vi "Sensor_Reads.vi"() -> ()   [LabVIEW 2019]
uses:
  M14 Hardware/Flywheel/M14_Flywheel_Hardware_Globals.vi
  M14 Hardware/Drive/M14_Drive_Hardware_Globals.vi
  M14 Hardware/Spindexer/M14_Hardware_Spindexer_Globals.vi
  M14 Hardware/New Magazine/New_Magazine_Hardware_Globals.vi
  M14 Hardware/Turret/M14 Turret_Hardware_Globals.vi
  M14 Hardware/Control Panel/M14_Control_Panel_Globals.vi
  Subsystems/Sensing/Sensor_Values.vi
  <vilib>/Rock Robotics/WPI/ThirdParty/Phoenix-LabVIEW/Motor Controller/Get/CTRE_Phoenix_MotorController_GetSelectedSensorData.vi
  M14 Hardware/Sensors/IMU/M14_IMU_Hardware_Globals.vi
  M14 Hardware/Sensors/IRs & Limits/M14_IR&Limits_Hardware_Globals.vi
  <vilib>/Rock Robotics/WPI/ThirdParty/Phoenix-LabVIEW/Pigeon IMU/CTRE_PigeonIMU_GetYPR.vi
panel:
  out "Right_Drive_Position(feet)":dbl
  out "Left_Drive_Position(feet)":dbl
  in  "F":dbl=0.365
  in  "D":dbl
  in  "I":dbl
  in  "P":dbl
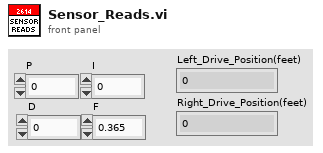
[diagram p1: front panel]
types:
  T1 = typedef "WPI_MotorControlDeviceRef.ctl" = cluster{"DeviceStatus":errorcluster, "Type":T2, "PWM":cluster{"PWM Channel":T3, "DeadBand":T4}, "CAN":cluster{"Device Number":u8, "SetOutput VI Ref":variant, "GetOutput VI Ref":variant, "Enable VI Ref":variant, "Disable VI Ref":variant, "Data":variant}, "Invert":bool, "DIO PWM":cluster{"PWM \"Enable\" Channel":T3, "DIOChannel":T5, "PWM Rate":dbl}}
  T2 = typedef "WPI_MotorControlType.ctl" = enum16{"PWM", "CAN", "DIO PWM"}
  T3 = typedef "FPGA_DIOPWMChannel.ctl" = enum8{"PWM 0", "PWM 1", "PWM 2", "PWM 3", "PWM 4", "PWM 5", "PWM 6", "PWM 7", "PWM 8", "PWM 9", "PWM MXP 0", "PWM MXP 1", "PWM MXP 2", "PWM MXP 3", "PWM MXP 4", "PWM MXP 5", "PWM MXP 6", "PWM MXP 7", "PWM MXP 8", "PWM MXP 9", "Invalid"}
  T4 = typedef "WPI_PWMDeadband.ctl" = cluster{"Name":string, "maxPositivePwm":i32, "minPositivePwm":i32, "centerPwm":i32, "maxNegativePwm":i32, "minNegativePwm":i32, "angularRange":u16}
  T5 = typedef "FPGA_DIOChannel.ctl" = enum8{"DIO 0", "DIO 1", "DIO 2", "DIO 3", "DIO 4", "DIO 5", "DIO 6", "DIO 7", "DIO 8", "DIO 9", "DIO MXP 0", "DIO MXP 1", "DIO MXP 2", "DIO MXP 3", "DIO MXP 4", "DIO MXP 5", "DIO MXP 6", "DIO MXP 7", "DIO MXP 8", "DIO MXP 9", "DIO MXP 10", "DIO MXP 11", "DIO MXP 12", "DIO MXP 13", "DIO MXP 14", "DIO MXP 15", "SPI Port CS1", "SPI Port CS2", "SPI Port CS3", "SPI Port MISO", "SPI Port MOSI", "Invalid"}
  T6 = typedef "CTRE_PigeonIMU_DeviceRef.ctl" = cluster{"DeviceStatus":errorcluster, "Device Number":u8, "Type":T7, "Device ID":u32, "Handle":u64, "UsageFrame":u32, "Library Path":path}
  T7 = typedef "CTRE_PigeonIMU_ConnectionType.ctl" = u32
  T8 = typedef "WPI_DigitalInputDevRef.ctl" = cluster{"DevStatus":errorcluster, "DIO Channel":T5}
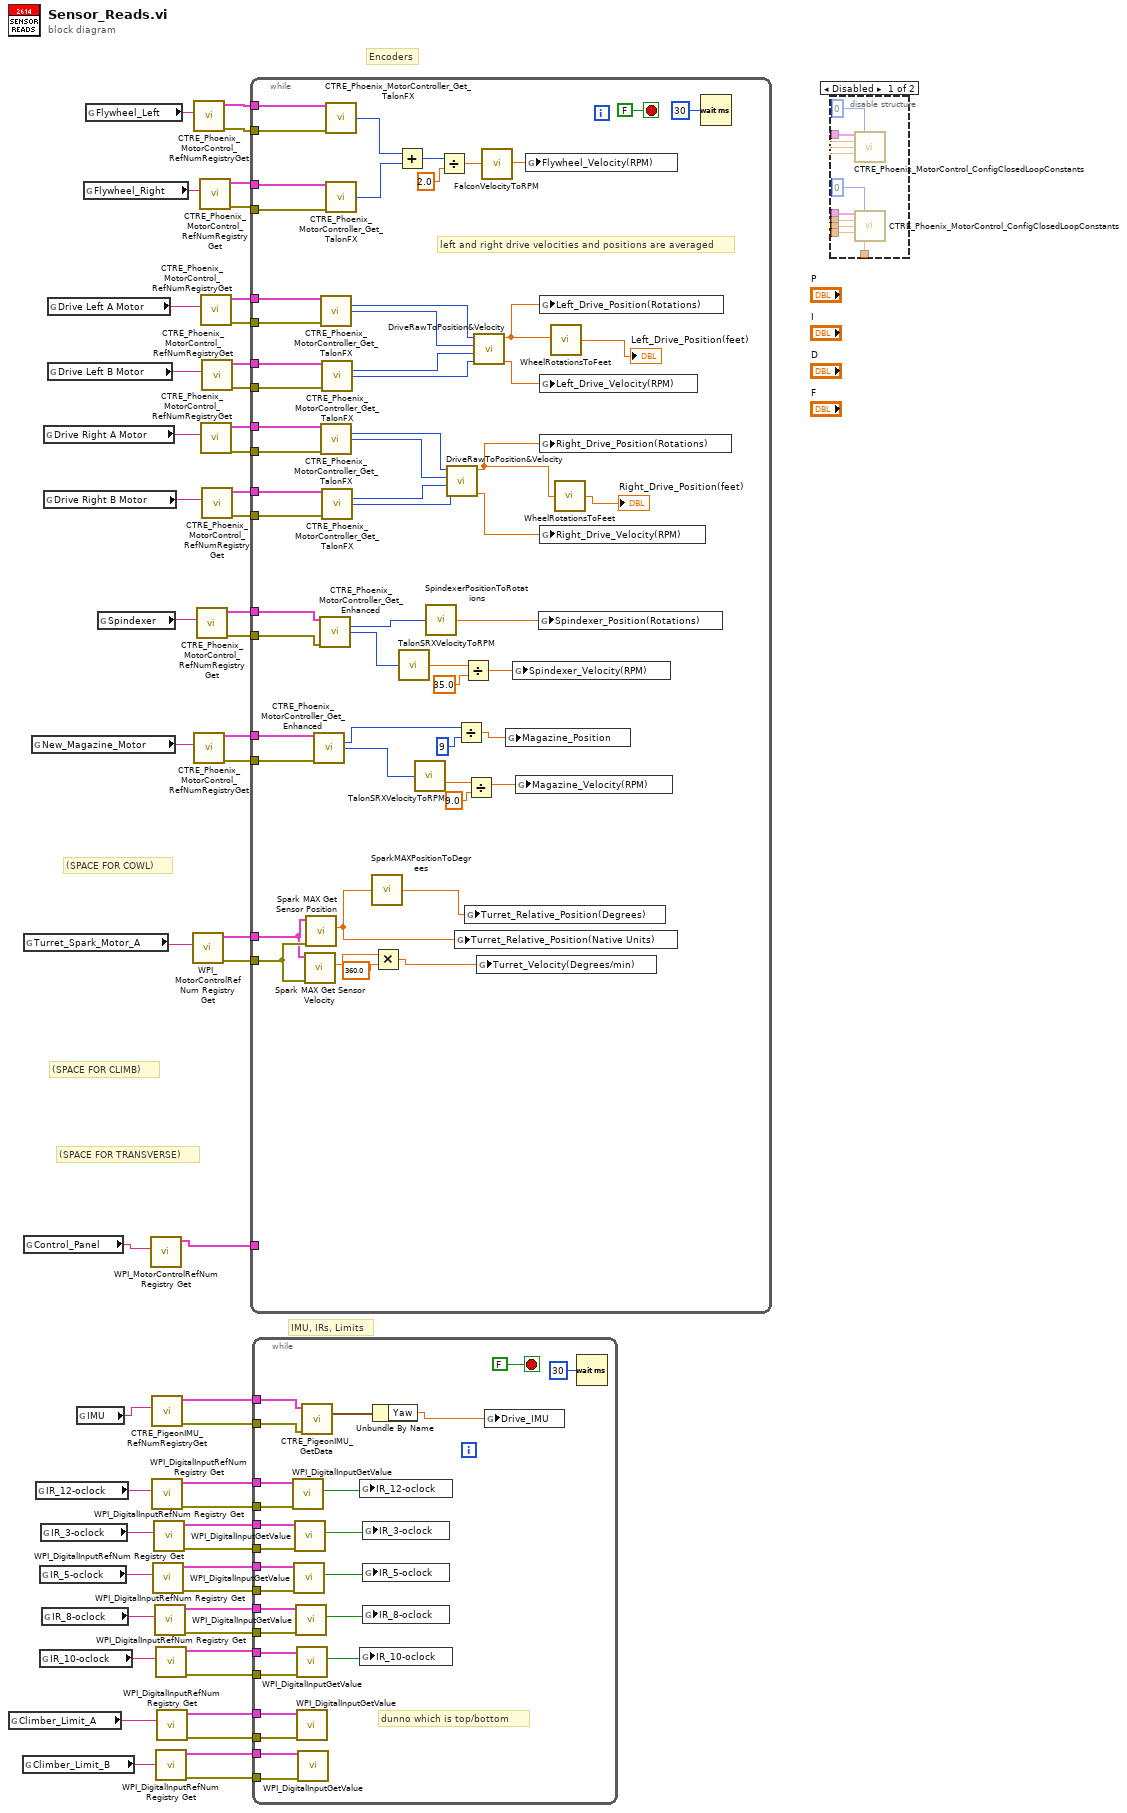
[diagram p0: block diagram]
diagram:
  # "IMU, IRs, Limits"
  # "(SPACE FOR TRANSVERSE)"
  # "(SPACE FOR CLIMB)"
  # "(SPACE FOR COWL)"
  # "Encoders"
  n1 = global read "M14_IR&Limits_Hardware_Globals.vi" "Climber_Limit_A"() -> (w6:string)
  n2 = global read "M14_IR&Limits_Hardware_Globals.vi" "Climber_Limit_B"() -> (w5:string)
  n3 = global read "M14 Turret_Hardware_Globals.vi" "Turret_Spark_Motor_A"() -> (w35:string)
  n4 = global read "M14_Control_Panel_Globals.vi" "Control_Panel"() -> (w33:string)
  n5 = global read "New_Magazine_Hardware_Globals.vi" "New_Magazine_Motor"() -> (w37:string)
  n6 = global read "M14_IR&Limits_Hardware_Globals.vi" "IR_12-oclock"() -> (w19:string)
  n7 = global read "M14_IR&Limits_Hardware_Globals.vi" "IR_5-oclock"() -> (w13:string)
  n8 = global read "M14_IR&Limits_Hardware_Globals.vi" "IR_10-oclock"() -> (w7:string)
  n9 = global read "M14_IR&Limits_Hardware_Globals.vi" "IR_3-oclock"() -> (w18:string)
  n10 = global read "M14_IR&Limits_Hardware_Globals.vi" "IR_8-oclock"() -> (w12:string)
  n11 = global read "M14_Drive_Hardware_Globals.vi" "Drive Right A Motor"() -> (w40:string)
  n12 = global read "M14_Drive_Hardware_Globals.vi" "Drive Right B Motor"() -> (w43:string)
  n13 = global read "M14_Drive_Hardware_Globals.vi" "Drive Left A Motor"() -> (w47:string)
  n14 = global read "M14_Drive_Hardware_Globals.vi" "Drive Left B Motor"() -> (w44:string)
  n15 = global read "M14_IMU_Hardware_Globals.vi" "IMU"() -> (w31:string)
  n16 = global read "M14_Flywheel_Hardware_Globals.vi" "Flywheel_Right"() -> (w52:string)
  n17 = global read "M14_Flywheel_Hardware_Globals.vi" "Flywheel_Left"() -> (w53:string)
  n18 = global read "M14_Hardware_Spindexer_Globals.vi" "Spindexer"() -> (w39:string)
  n19 = call <vilib>:"WPI_MotorControlRefNum Registry Get.vi"("refnum name"=w33) -> ("MotorControlDevRef"=w32:T1)  [unwired: 9 in, 1 out]
  n20 = call <vilib>:"CTRE_PigeonIMU_RefNumRegistryGet.vi"("refnum name"=w31) -> ("error out"=w22:errorcluster, "PigeonIMUDevRef"=w30:T6)  [unwired: 9 in]
  n21 = call <vilib>:"WPI_DigitalInputRefNum Registry Get.vi"("refnum name"=w19) -> ("error out"=w20:errorcluster, "DigitalInputDevRef"=w21:T8)  [unwired: 9 in]
  n22 = call <vilib>:"WPI_DigitalInputRefNum Registry Get.vi"("refnum name"=w13) -> ("error out"=w14:errorcluster, "DigitalInputDevRef"=w15:T8)  [unwired: 9 in]
  n23 = call <vilib>:"WPI_DigitalInputRefNum Registry Get.vi"("refnum name"=w18) -> ("error out"=w17:errorcluster, "DigitalInputDevRef"=w16:T8)  [unwired: 9 in]
  n24 = call <vilib>:"WPI_DigitalInputRefNum Registry Get.vi"("refnum name"=w12) -> ("error out"=w11:errorcluster, "DigitalInputDevRef"=w10:T8)  [unwired: 9 in]
  n25 = call <vilib>:"WPI_DigitalInputRefNum Registry Get.vi"("refnum name"=w7) -> ("error out"=w8:errorcluster, "DigitalInputDevRef"=w9:T8)  [unwired: 9 in]
  n26 = call <vilib>:"WPI_DigitalInputRefNum Registry Get.vi"("refnum name"=w5) -> ("error out"=w1:errorcluster, "DigitalInputDevRef"=w2:T8)  [unwired: 9 in]
  n27 = call <vilib>:"WPI_DigitalInputRefNum Registry Get.vi"("refnum name"=w6) -> ("error out"=w3:errorcluster, "DigitalInputDevRef"=w4:T8)  [unwired: 9 in]
  n28 = call <vilib>:"WPI_MotorControlRefNum Registry Get.vi"("refnum name"=w35) -> ("error out"=w23:errorcluster, "MotorControlDevRef"=w34:T1)  [unwired: 9 in]
  n29 = call <vilib>:"CTRE_Phoenix_MotorControl_RefNumRegistryGet.vi"("refnum name"=w53) -> ("error out"=w50:errorcluster, "PhoenixMotorControlDevRef"=w51:T1)  [unwired: 9 in]
  n30 = call <vilib>:"CTRE_Phoenix_MotorControl_RefNumRegistryGet.vi"("refnum name"=w37) -> ("error out"=w24:errorcluster, "PhoenixMotorControlDevRef"=w36:T1)  [unwired: 9 in]
  n31 = call <vilib>:"CTRE_Phoenix_MotorControl_RefNumRegistryGet.vi"("refnum name"=w39) -> ("error out"=w25:errorcluster, "PhoenixMotorControlDevRef"=w38:T1)  [unwired: 9 in]
  n32 = call <vilib>:"CTRE_Phoenix_MotorControl_RefNumRegistryGet.vi"("refnum name"=w52) -> ("error out"=w48:errorcluster, "PhoenixMotorControlDevRef"=w49:T1)  [unwired: 9 in]
  n33 = call <vilib>:"CTRE_Phoenix_MotorControl_RefNumRegistryGet.vi"("refnum name"=w47) -> ("error out"=w29:errorcluster, "PhoenixMotorControlDevRef"=w46:T1)  [unwired: 9 in]
  n34 = call <vilib>:"CTRE_Phoenix_MotorControl_RefNumRegistryGet.vi"("refnum name"=w40) -> ("error out"=w27:errorcluster, "PhoenixMotorControlDevRef"=w41:T1)  [unwired: 9 in]
  n35 = call <vilib>:"CTRE_Phoenix_MotorControl_RefNumRegistryGet.vi"("refnum name"=w44) -> ("error out"=w28:errorcluster, "PhoenixMotorControlDevRef"=w45:T1)  [unwired: 9 in]
  n36 = call <vilib>:"CTRE_Phoenix_MotorControl_RefNumRegistryGet.vi"("refnum name"=w43) -> ("error out"=w26:errorcluster, "PhoenixMotorControlDevRef"=w42:T1)  [unwired: 9 in]
  n37 = while {
    tunnel: w51 -> [w109]
    tunnel: w50 -> [w108]
    tunnel: w49 -> [w107]
    tunnel: w48 -> [w106]
    tunnel: w46 -> [w105]
    tunnel: w45 -> [w104]
    tunnel: w41 -> [w102]
    tunnel: w42 -> [w103]
    tunnel: w38 -> [w92]
    tunnel: w36 -> [w89]
    tunnel: w34 -> [w70]
    tunnel: w32 -> [_]
    tunnel: w29 -> [w77]
    tunnel: w28 -> [w76]
    tunnel: w27 -> [w75]
    tunnel: w26 -> [w74]
    tunnel: w25 -> [w73]
    tunnel: w24 -> [w72]
    tunnel: w23 -> [w71]
    stop <- FALSE stop-if-true
    # "left and right drive velocities and positions are averaged"
    n38 = call <vilib>:"Spark MAX Get Sensor Velocity.vi"("error in (no error)"=w71, "MotorControlDevRef in"=w70) -> ("Sensor Velocity"=w61:dbl)  [unwired: 6 in, 3 out]
    n39 = call <vilib>:"Spark MAX Get Sensor Position.vi"("error in (no error)"=w71, "MotorControlDevRef in"=w70) -> ("Sensor Position"=w58:dbl)  [unwired: 6 in, 3 out]
    n40 = call-poly <vilib>:"CTRE_Phoenix_MotorController_Get_Enhanced.vi"("PhoenixMotorControlDevRef"=w89, "error in"=w72) -> ("Position (Raw Sensor Units)"=w85:i32, "Velocity (Raw Sensor Units per 100 ms)"=w88:i32)  [unwired: 10 in, 2 out]
    n41 = call-poly <vilib>:"CTRE_Phoenix_MotorController_Get_Enhanced.vi"("PhoenixMotorControlDevRef"=w92, "error in"=w73) -> ("Position (Raw Sensor Units)"=w90:i32, "Velocity (Raw Sensor Units per 100 ms)"=w91:i32)  [unwired: 10 in, 2 out]
    n42 = call-poly <vilib>:"CTRE_Phoenix_MotorController_Get_TalonFX.vi"("PhoenixMotorControlDevRef"=w105, "error in"=w77) -> ("Position (Raw Sensor Units)"=w94:i32, "Velocity (Raw Sensor Units per 100 ms)"=w101:i32)  [unwired: 10 in, 2 out]
    n43 = call-poly <vilib>:"CTRE_Phoenix_MotorController_Get_TalonFX.vi"("PhoenixMotorControlDevRef"=w102, "error in"=w75) -> ("Position (Raw Sensor Units)"=w67:i32, "Velocity (Raw Sensor Units per 100 ms)"=w66:i32)  [unwired: 10 in, 2 out]
    n44 = call-poly <vilib>:"CTRE_Phoenix_MotorController_Get_TalonFX.vi"("PhoenixMotorControlDevRef"=w104, "error in"=w76) -> ("Position (Raw Sensor Units)"=w93:i32, "Velocity (Raw Sensor Units per 100 ms)"=w69:i32)  [unwired: 10 in, 2 out]
    n45 = call-poly <vilib>:"CTRE_Phoenix_MotorController_Get_TalonFX.vi"("PhoenixMotorControlDevRef"=w103, "error in"=w74) -> ("Position (Raw Sensor Units)"=w65:i32, "Velocity (Raw Sensor Units per 100 ms)"=w64:i32)  [unwired: 10 in, 2 out]
    n46 = call-poly <vilib>:"CTRE_Phoenix_MotorController_Get_TalonFX.vi"("PhoenixMotorControlDevRef"=w109, "error in"=w108) -> ("Velocity (Raw Sensor Units per 100 ms)"=w97:i32)  [unwired: 10 in, 3 out]
    n47 = call-poly <vilib>:"CTRE_Phoenix_MotorController_Get_TalonFX.vi"("PhoenixMotorControlDevRef"=w107, "error in"=w106) -> ("Velocity (Raw Sensor Units per 100 ms)"=w96:i32)  [unwired: 10 in, 3 out]
    n48 = call "SparkMAXPositionToDegrees.vi"("Sensor Position"=w58) -> ("degrees"=w59:dbl)  [unwired: 4 in]
    n49 = Multiply(x=w61, y=360.0) -> (x*y=w62:dbl)
    n50 = Add(x=w97, y=w96) -> (x+y=w98:i32)
    n51 = call "TalonSRXVelocityToRPM.vi"("Velocity (Raw Sensor Units per 100 ms)"=w91) -> ("RPM"=w81:dbl)  [unwired: 4 in]
    n52 = call "TalonSRXVelocityToRPM.vi"("Velocity (Raw Sensor Units per 100 ms)"=w88) -> ("RPM"=w87:dbl)  [unwired: 4 in]
    n53 = call "SpindexerPositionToRotations.vi"("Position (Raw Sensor Units)"=w90) -> ("Numeric"=w78:dbl)  [unwired: 4 in]
    n54 = Divide(x=w98, y=2.0) -> (x/y=w95:dbl)
    n55 = call "DriveRawToPosition&Velocity.vi"("Velocity (Raw Sensor Units per 100 ms) B"=w64, "Position (Raw Sensor Units) B"=w65, "Velocity (Raw Sensor Units per 100 ms) A"=w66, "Position (Raw Sensor Units) A"=w67) -> ("Velocity"=w63:dbl, "Position"=w55:dbl)  [unwired: 6 in]
    n56 = global write "Sensor_Values.vi" "Turret_Relative_Position(Native Units)"(w58) -> ()
    n57 = Divide(x=w85, y=9) -> (x/y=w86:dbl)
    n58 = Divide(x=w81, y=35.0) -> (x/y=w79:dbl)
    n59 = global write "Sensor_Values.vi" "Turret_Relative_Position(Degrees)"(w59) -> ()
    n60 = Divide(x=w87, y=9.0) -> (x/y=w83:dbl)
    n61 = call "DriveRawToPosition&Velocity.vi"("Velocity (Raw Sensor Units per 100 ms) B"=w69, "Position (Raw Sensor Units) B"=w93, "Velocity (Raw Sensor Units per 100 ms) A"=w101, "Position (Raw Sensor Units) A"=w94) -> ("Velocity"=w68:dbl, "Position"=w57:dbl)  [unwired: 6 in]
    n62 = global write "Sensor_Values.vi" "Turret_Velocity(Degrees/min)"(w62) -> ()
    n63 = call "FalconVelocityToRPM.vi"("raw sensor units / 100 ms"=w95) -> ("RPM"=w100:dbl)  [unwired: 4 in]
    n64 = global write "Sensor_Values.vi" "Magazine_Position"(w86) -> ()
    n65 = global write "Sensor_Values.vi" "Spindexer_Velocity(RPM)"(w79) -> ()
    n66 = global write "Sensor_Values.vi" "Magazine_Velocity(RPM)"(w83) -> ()
    n67 = global write "Sensor_Values.vi" "Flywheel_Velocity(RPM)"(w100) -> ()
    n68 = global write "Sensor_Values.vi" "Spindexer_Position(Rotations)"(w78) -> ()
    n69 = global write "Sensor_Values.vi" "Left_Drive_Position(Rotations)"(w57) -> ()
    n70 = global write "Sensor_Values.vi" "Left_Drive_Velocity(RPM)"(w68) -> ()
    n71 = global write "Sensor_Values.vi" "Right_Drive_Position(Rotations)"(w55) -> ()
    n72 = global write "Sensor_Values.vi" "Right_Drive_Velocity(RPM)"(w63) -> ()
    n73 = call "WheelRotationsToFeet.vi"("rotations"=w57) -> ("feet"=→"Left_Drive_Position(feet)":dbl)  [unwired: 4 in]
    n74 = call "WheelRotationsToFeet.vi"("rotations"=w55) -> ("feet"=→"Right_Drive_Position(feet)":dbl)  [unwired: 4 in]
    n75 = Wait (ms)(milliseconds to wait=u32 30) -> ()  [unwired: 1 out]
  }
  n76 = while {
    tunnel: w30 -> [w135]
    tunnel: w22 -> [w134]
    tunnel: w21 -> [w130]
    tunnel: w20 -> [w129]
    tunnel: w16 -> [w127]
    tunnel: w17 -> [w128]
    tunnel: w15 -> [w126]
    tunnel: w14 -> [w125]
    tunnel: w10 -> [w123]
    tunnel: w11 -> [w124]
    tunnel: w9 -> [w122]
    tunnel: w8 -> [w121]
    tunnel: w4 -> [w115]
    tunnel: w3 -> [w114]
    tunnel: w2 -> [w113]
    tunnel: w1 -> [w112]
    stop <- FALSE stop-if-true
    # "dunno which is top/bottom"
    n77 = call <vilib>:"WPI_DigitalInputGetValue.vi"("error in (no error)"=w129, "DigitalInputDevRef"=w130) -> ("Value"=w120:bool)  [unwired: 7 in, 2 out]
    n78 = call <vilib>:"WPI_DigitalInputGetValue.vi"("error in (no error)"=w125, "DigitalInputDevRef"=w126) -> ("Value"=w118:bool)  [unwired: 7 in, 2 out]
    n79 = call <vilib>:"WPI_DigitalInputGetValue.vi"("error in (no error)"=w128, "DigitalInputDevRef"=w127) -> ("Value"=w119:bool)  [unwired: 7 in, 2 out]
    n80 = call <vilib>:"WPI_DigitalInputGetValue.vi"("error in (no error)"=w124, "DigitalInputDevRef"=w123) -> ("Value"=w117:bool)  [unwired: 7 in, 2 out]
    n81 = call <vilib>:"WPI_DigitalInputGetValue.vi"("error in (no error)"=w121, "DigitalInputDevRef"=w122) -> ("Value"=w116:bool)  [unwired: 7 in, 2 out]
    n82 = call <vilib>:"WPI_DigitalInputGetValue.vi"("error in (no error)"=w114, "DigitalInputDevRef"=w115) -> ()  [unwired: 7 in, 3 out]
    n83 = call <vilib>:"WPI_DigitalInputGetValue.vi"("error in (no error)"=w112, "DigitalInputDevRef"=w113) -> ()  [unwired: 7 in, 3 out]
    n84 = call-poly <vilib>:"CTRE_PigeonIMU_GetData.vi"("error in (no error)"=w134, "PigeonIMUDevRef"=w135) -> ("Yaw Pitch Roll"=w133:cluster{"Yaw":dbl, "Pitch":dbl, "Roll":dbl})  [unwired: 7 in, 2 out]
    n85 = global write "Sensor_Values.vi" "IR_12-oclock"(w120) -> ()
    n86 = global write "Sensor_Values.vi" "IR_10-oclock"(w116) -> ()
    n87 = global write "Sensor_Values.vi" "IR_3-oclock"(w119) -> ()
    n88 = global write "Sensor_Values.vi" "IR_5-oclock"(w118) -> ()
    n89 = global write "Sensor_Values.vi" "IR_8-oclock"(w117) -> ()
    n90 = Unbundle By Name(w133) -> ("Yaw"=w132:dbl)
    n91 = global write "Sensor_Values.vi" "Drive_IMU"(w132) -> ()
    n92 = Wait (ms)(milliseconds to wait=u32 30) -> ()  [unwired: 1 out]
  }
  n93 = disable-structure shown="Disabled" {
    disable-tunnel: _ -> [w144 _]
    disable-tunnel: _ -> [w143 _]
    disable-tunnel: _ -> [w142 _]
    disable-tunnel: _ -> [w141 _]
    disable-tunnel: _ -> [w140 _]
    disable-tunnel: _ -> [w139 _]
    frame Disabled {
      n94 = call <vilib>:"CTRE_Phoenix_MotorControl_ConfigClosedLoopConstants.vi"("PhoenixMotorControlDevRef"=w143, "slotIdx"=0, "P"=w141, "I"=w140, "D"=w139) -> ()  [unwired: 9 in, 2 out]
      n95 = call <vilib>:"CTRE_Phoenix_MotorControl_ConfigClosedLoopConstants.vi"("PhoenixMotorControlDevRef"=w144, "slotIdx"=0, "P"=w141, "I"=w140, "D"=w139, "F"=w142) -> ()  [unwired: 8 in, 2 out]
    }
    frame Enabled {
    }
  }
